vi "EKG Monitor2.vi"() -> ()   [LabVIEW 2010]
uses:
  <instrlib>/niHWS/nihws.llb/niHWS Open File Permissions ID.ctl
  <vilib>/DAQmx/read.llb/DAQmx Read (Analog 1D Wfm NChan NSamp).vi
  <vilib>/DAQmx/create/channels.llb/DAQmx Create Channel (AI-Voltage-Basic).vi
  <vilib>/DAQmx/configure/timing.llb/DAQmx Timing (Sample Clock).vi
  Fear Conditioning/GlobalFear.vi
  <instrlib>/niHWS/nihws.llb/niHWS Write Digital U32.vi
  <instrlib>/niHWS/nihws.llb/niHWS Write Analog DBL.vi
  <instrlib>/niHWS/nihws.llb/niHWS Write Analog WDT.vi
  <vilib>/measure/matone.llb/Extract Single Tone Information N Chan.vi
  <vilib>/daqmx/miscellaneous.llb/DAQmx Fill In Error Info.vi
  Program Files (x86)/National Instruments/LabVIEW 2010/resource/objmgr/daqmx.rc
  <vilib>/measure/NI_MAPro.lvlib
panel:
  out "det Freq":dbl
  out "RAW ECG Signal":waveform(dbl)[](graph)
  in  "# average":dbl=20.0
  out "Shock":bool
  out "Audio":bool
  in  "DPI":dbl=350.0
  out "Cycles \ncompleted":dbl
  in  "stop 2":bool
  in  "Start":bool
  in  "Rate Corrector":bool=TRUE
  out "Skipped":bool
  out "Error Thr":dbl
  out "Threshold":dbl
  in  "HR % Change\nThreshold":dbl(slide)=25.0 scale=0.0..25.0
  out "Detected HR":dynamicdata(graph)
  in  "Mouse Axis":bool
  out "Activity monitor":dynamicdata(graph)
  in  "Activity mouse":refnum<visa-resource-name>
  out "HR":dbl format="%#_4g"
  out "HR":dbl(graph)
  out "Filtered ECG Signal":waveform(dbl)[](graph)
  in  "Recording Path":path
  in  "Record":bool
  in  "stop":bool
  in  "Recording channels":tag
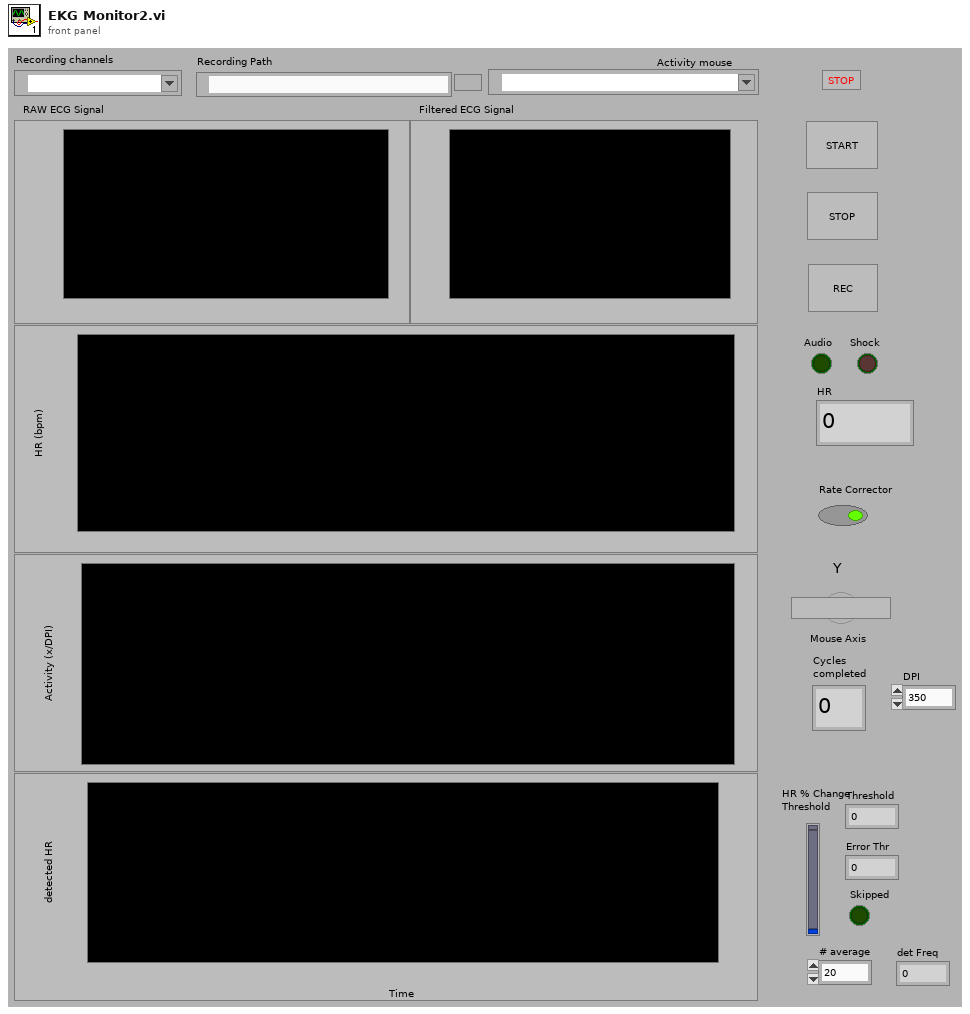
[diagram p1: front panel]
types:
  T1 = typedef "niHWS Open File Permissions ID.ctl" = enum32{"Read Only", "Read/Write Existing", "Read/Write/Create New", "Read/Write/Create New Always"}
  T2 = cluster{"approx freq. (optional)":dbl, "search (+/- % of Fsampl.)":dbl}
  T3 = cluster{"Array":dbl[], "Array 2":dbl[], "Array 3":dbl[], "Array 4":dbl[], "Array 5":dbl[], "Array 6":dbl[], "Array 7":dbl[], "Array 8":dbl[]}
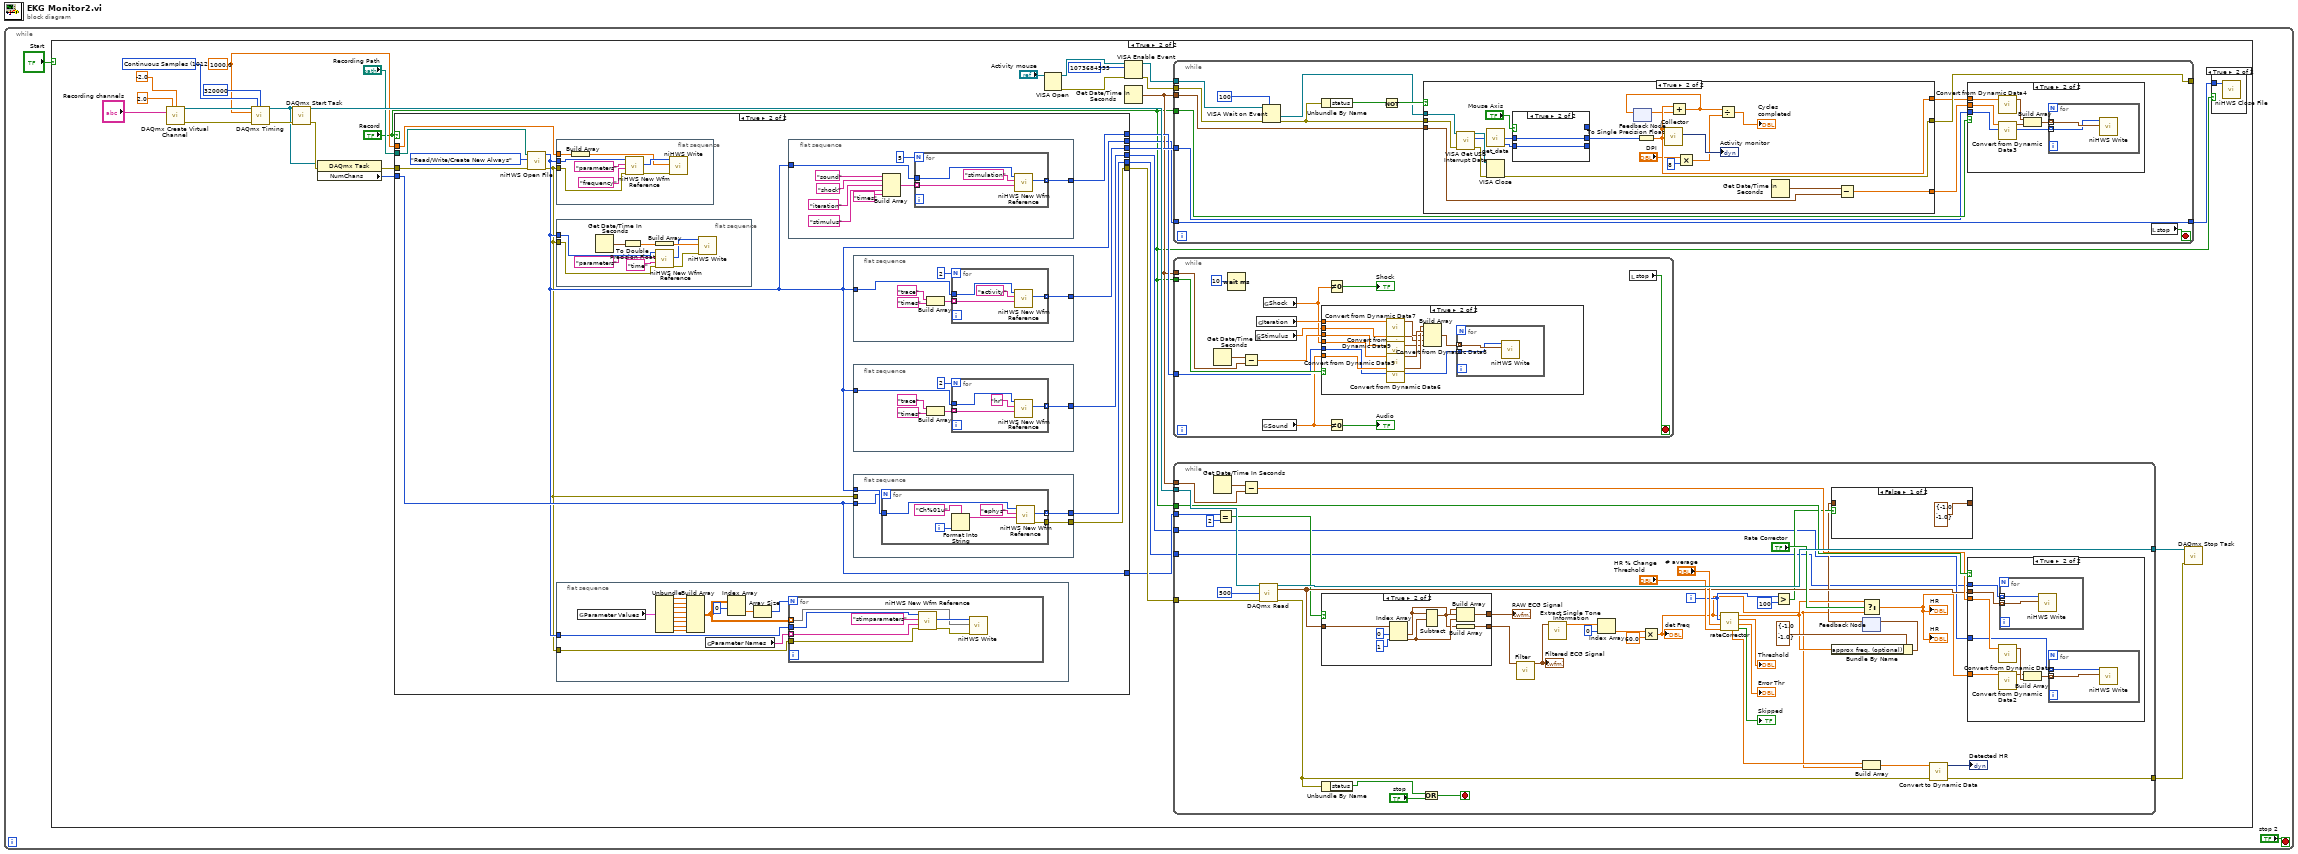
[diagram p0: block diagram]
diagram:
  n1 = while {
    stop <- "stop 2" stop-if-true
    n2 = case shown="True" "Start" {
      frame False {
      }
      frame True {
        w31 = 10123 items=["Finite Samples"=10178, "Continuous Samples"=10123, "Hardware Timed Single Point"=12522] ("sample mode")
        w5 = 1000.0 ("rate")
        n3 = call-poly <vilib>:"DAQmx Create Virtual Channel.vi"("maximum value"=2.0, "minimum value"=-2.0, "physical channels"="Recording channels") -> ("task out"=w32:refnum<k21>, "error out"=w29:errorcluster)  [unwired: 11 in]
        n4 = call-poly <vilib>:"DAQmx Timing.vi"("task/channels in"=w32, "sample mode"=w31, "samples per channel"=320000, "rate"=w5, "error in"=w29) -> ("task out"=w19:refnum<k21>, "error out"=w28:errorcluster)  [unwired: 9 in]
        n5 = call <vilib>:"DAQmx Start Task.vi"("task/channels in"=w19, "error in"=w28) -> ("task out"=w27:refnum<k21>, "error out"=w22:errorcluster)  [unwired: 12 in]
        n6 = property class="DAQmx Task"(reference=w19, error in=w22) -> (error out=w21:errorcluster, "NumChans"=w24:u32)  [unwired: 1 out]
        n7 = case shown="True" "Record" {
          tunnel: w24 -> [w113 w121]
          tunnel: "Recording Path" -> [_ w126]
          tunnel: [w114 w115] -> w20
          tunnel: w21 -> [w114 w124]
          tunnel: [_ w123] -> w12
          tunnel: [_ w122] -> w11
          tunnel: [_ w118] -> w9
          tunnel: [w113 w121] -> w7
          tunnel: [_ w120] -> w6
          tunnel: w5 -> [_ w119]
          tunnel: [_ w116] -> w4
          frame False {
          }
          frame True {
            n8 = call <instrlib>:"niHWS Open File.vi"("error in (no error)"=w124, "permissions (0:read only)"=niHWS_Open_File_Permissions_ID."Read/Write/Create New Always", "file path"=w126) -> ("error out"=w117:errorcluster, "file handle"=w118:u32)  [unwired: 7 in]
            n9 = flat-sequence {
              tunnel: w119 -> [w183]
              tunnel: w117 -> [w182]
              tunnel: w118 -> [w181]
              frame #0 {
                n10 = Build Array(w183) -> (w184:dbl[])
                n11 = call <instrlib>:"niHWS New Wfm Reference.vi"("error in (no error)"=w182, "waveform name (empty)"="frequency" ("group name (empty)"), "group name (empty)"="parameters", "file handle in"=w181) -> ("error out"=w180:errorcluster, "waveform reference"=w187:u32)  [unwired: 5 in, 1 out]
                n12 = call-poly <instrlib>:"niHWS Write.vi"("error in (no error)"=w180, "data"=w184, "waveform reference in"=w187) -> ()  [unwired: 7 in, 2 out]
              }
            }
            n13 = flat-sequence {
              tunnel: w117 -> [w179]
              tunnel: w118 -> [w178]
              frame #0 {
                n14 = Get Date/Time In Seconds() -> (seconds since 1Jan1904=w177:timestamp)
                n15 = To Double Precision Float(number=w177) -> (double precision float=w176:dbl)
                n16 = Build Array(w176) -> (w175:dbl[])
                n17 = call <instrlib>:"niHWS New Wfm Reference.vi"("error in (no error)"=w179, "waveform name (empty)"="time" ("group name (empty)"), "group name (empty)"="parameters", "file handle in"=w178) -> ("error out"=w171:errorcluster, "waveform reference"=w172:u32)  [unwired: 5 in, 1 out]
                n18 = call-poly <instrlib>:"niHWS Write.vi"("error in (no error)"=w171, "data"=w175, "waveform reference in"=w172) -> ()  [unwired: 7 in, 2 out]
              }
            }
            n19 = flat-sequence {
              tunnel: w118 -> [w189]
              tunnel: w117 -> [w188]
              frame #0 {
                n20 = global read "GlobalFear.vi" "Parameter Values"() -> (w190:T3)
                n21 = Unbundle(w190) -> ("Array"=w191:dbl[], "Array 2"=w192:dbl[], "Array 3"=w193:dbl[], "Array 4"=w194:dbl[], "Array 5"=w195:dbl[], "Array 6"=w196:dbl[], "Array 7"=w197:dbl[], "Array 8"=w198:dbl[])
                n22 = Build Array(w191, w192, w193, w194, w195, w196, w197, w198) -> (w202:dbl[][])
                n23 = global read "GlobalFear.vi" "Parameter Names"() -> (w203:string[])
                n24 = Index Array(array=w202, index (row)=0) -> (element=w200:dbl[])  [unwired: 1 in]
                n25 = Array Size(array=w200) -> (size(s)=w199:i32)
                n26 = for {
                  N: w199 -> [_]
                  tunnel: w202 -> [w208] mode=indexing
                  tunnel: w203 -> [w207] mode=indexing
                  tunnel: w189 -> [w206]
                  tunnel: w188 -> [w205]
                  n27 = call <instrlib>:"niHWS New Wfm Reference.vi"("error in (no error)"=w205, "waveform name (empty)"=w207, "group name (empty)"="stimparameters", "file handle in"=w206) -> ("error out"=w204:errorcluster, "waveform reference"=w209:u32)  [unwired: 5 in, 1 out]
                  n28 = call-poly <instrlib>:"niHWS Write.vi"("error in (no error)"=w204, "data"=w208, "waveform reference in"=w209) -> ()  [unwired: 7 in, 2 out]
                }
              }
            }
            n29 = flat-sequence {
              tunnel: [w134] -> w122
              tunnel: w118 -> [w133]
              frame #0 {
                n30 = Build Array("sound" ("format string"), "shock" ("format string"), "iteration" ("format string"), "stimulus" ("format string"), "times") -> (w127:string[])
                n31 = for {
                  N: 5 -> [_]
                  tunnel: [w139] -> w134 mode=indexing
                  tunnel: w133 -> [w137]
                  tunnel: w127 -> [w136] mode=indexing
                  n32 = call <instrlib>:"niHWS New Wfm Reference.vi"("waveform name (empty)"=w136, "group name (empty)"="stimulation", "file handle in"=w137) -> ("waveform reference"=w139:u32)  [unwired: 6 in, 2 out]
                }
              }
            }
            n33 = flat-sequence {
              tunnel: [w155] -> w123
              tunnel: w118 -> [w154]
              frame #0 {
                n34 = Build Array("trace" ("format string"), "times" ("format string")) -> (w150:string[])
                n35 = for {
                  N: 2 -> [_]
                  tunnel: [w159] -> w155 mode=indexing
                  tunnel: w154 -> [w157]
                  tunnel: w150 -> [w156] mode=indexing
                  n36 = call <instrlib>:"niHWS New Wfm Reference.vi"("waveform name (empty)"=w156, "group name (empty)"="activity", "file handle in"=w157) -> ("waveform reference"=w159:u32)  [unwired: 6 in, 2 out]
                }
              }
            }
            n37 = flat-sequence {
              tunnel: [w144] -> w120
              tunnel: w118 -> [w143]
              frame #0 {
                n38 = Build Array("trace" ("format string"), "times" ("format string")) -> (w140:string[])
                n39 = for {
                  N: 2 -> [_]
                  tunnel: [w149] -> w144 mode=indexing
                  tunnel: w143 -> [w147]
                  tunnel: w140 -> [w146] mode=indexing
                  n40 = call <instrlib>:"niHWS New Wfm Reference.vi"("waveform name (empty)"=w146, "group name (empty)"="hr", "file handle in"=w147) -> ("waveform reference"=w149:u32)  [unwired: 6 in, 2 out]
                }
              }
            }
            n41 = flat-sequence {
              tunnel: w121 -> [w162]
              tunnel: w118 -> [w163]
              tunnel: w117 -> [_]
              tunnel: [w161] -> w116
              tunnel: [w160] -> w115
              frame #0 {
                n42 = for {
                  N: w162 -> [_]
                  tunnel: [w165] -> w161 mode=indexing
                  tunnel: [w164] -> w160
                  tunnel: w163 -> [w170]
                  i -> [w168]
                  n43 = Format Into String(format string="Ch%01u", w168) -> (resulting string=w166:string)  [unwired: 2 in, 1 out]
                  n44 = call <instrlib>:"niHWS New Wfm Reference.vi"("waveform name (empty)"=w166, "group name (empty)"="ephys", "file handle in"=w170) -> ("error out"=w164:errorcluster, "waveform reference"=w165:u32)  [unwired: 6 in, 1 out]
                }
              }
            }
          }
        }
        n45 = VISA Open(VISA resource name="Activity mouse") -> (VISA resource name=w18:refnum<visa-resource-name>, error out=w17:errorcluster)  [unwired: 1 in, 3 out]
        n46 = VISA Enable Event(8:w17, 10:u32 1073684535 ("event type"), 11:w18) -> (0:w14:errorcluster, 3:w15:refnum<visa-resource-name>)  [unwired: 1 out]
        n47 = Get Date/Time In Seconds() -> (seconds since 1Jan1904=w10:timestamp)
        n48 = while {
          tunnel: w15 -> [w77]
          tunnel: w14 -> [w76]
          tunnel: w10 -> [w75]
          tunnel: [w69] -> _
          tunnel: "Record" -> [w68]
          tunnel: w12 -> [w65]
          tunnel: w9 -> [w63]
          tunnel: [w63] -> w8
          stop <- w64 stop-if-true
          n49 = VISA Wait on Event(7:u32 100 ("timeout (0)"), 8:w76, 11:w77) -> (0:w70:errorcluster, 1:w71:refnum<visa-resource-name>)  [unwired: 4 out]
          n50 = Unbundle By Name(w70) -> ("status"=w72:bool)
          n51 = Not(x=w72) -> (.not. x?=w73:bool)
          n52 = case shown="True" w73 {
            tunnel: w71 -> [_ w104]
            tunnel: [w86 w103] -> w69
            tunnel: w70 -> [w86 w102]
            tunnel: w75 -> [_ w100]
            tunnel: [_ w93] -> w67
            tunnel: [_ w99] -> w66
            frame False {
            }
            frame True {
              n53 = call <vilib>:"VISA Get USB Interrupt Data.vi"("error in (no error)"=w102, "VISA USB Intr Event"=w104) -> ("error out"=w105:errorcluster, "data buffer"=w101:u8[], "VISA USB Intr Event out"=w106:refnum<visa-resource-name>)  [unwired: 7 out]
              n54 = call "get_data.vi"("data buffer"=w101) -> ("X Value"=w96:i8, "Y Value"=w94:i8)  [unwired: 1 out]
              n55 = VISA Close(VISA resource name=w106, error in (no error)=w105) -> (error out=w103:errorcluster)
              n56 = case shown="True" "Mouse Axis" {
                tunnel: w96 -> [w108 w111]
                tunnel: [w109 w111] -> w95
                tunnel: w94 -> [w109 w110]
                tunnel: [w108 _] -> _
                tunnel: [_ w110] -> _
                frame False {
                }
                frame True {
                }
              }
              n57 = feedback #1() -> (w92:sgl)  [unwired: 1 in]
              n58 = To Single Precision Float(number=w95) -> (single precision float=w93:sgl)
              n59 = call "Collector"("Signals"=w93) -> ("Collected Signals"=→"Activity monitor":dynamicdata)  [unwired: 9 in, 1 out]
              n60 = Add(x=w93, y=w92) -> (x+y=w90:sgl)
              n61 = feedback-in #1(w90) -> ()
              n62 = Multiply(x="DPI", y=8) -> (x*y=w91:dbl)
              n63 = Divide(x=w90, y=w91) -> (x/y=→"Cycles \ncompleted":dbl)
              n64 = Get Date/Time In Seconds() -> (seconds since 1Jan1904=w107:timestamp)
              n65 = Subtract(x=w107, y=w100) -> (x-y=w99:dbl)
            }
          }
          n66 = case shown="True" w68 {
            tunnel: w67 -> [_ w80]
            tunnel: w66 -> [_ w79]
            tunnel: w65 -> [_ w78]
            frame False {
            }
            frame True {
              n67 = call "Convert from Dynamic Data4"("Dynamic Data Type"=w80) -> ("Waveform"=w81:waveform(dbl))  [unwired: 3 in]
              n68 = call "Convert from Dynamic Data3"("Dynamic Data Type"=w79) -> ("Waveform"=w82:waveform(dbl))  [unwired: 3 in]
              n69 = Build Array(w81, w82) -> (w83:waveform(dbl)[])
              n70 = for {
                tunnel: w83 -> [w85] mode=indexing
                tunnel: w78 -> [w84] mode=indexing
                n71 = call-poly <instrlib>:"niHWS Write.vi"("analog waveform"=w85, "waveform reference in"=w84) -> ()  [unwired: 8 in, 2 out]
              }
            }
          }
          n72 = local read "stop"() -> (w64:bool)
        }
        n73 = while {
          tunnel: "Record" -> [w47]
          tunnel: w11 -> [w46]
          tunnel: w10 -> [w44]
          stop <- w48 stop-if-true
          n74 = Get Date/Time In Seconds() -> (seconds since 1Jan1904=w45:timestamp)
          n75 = Wait (ms)(milliseconds to wait=10) -> ()  [unwired: 1 out]
          n76 = Subtract(x=w45, y=w44) -> (x-y=w43:dbl)
          n77 = global read "GlobalFear.vi" "Stimulus"() -> (w36:dbl)
          n78 = global read "GlobalFear.vi" "Iteration"() -> (w42:dbl)
          n79 = global read "GlobalFear.vi" "Sound"() -> (w41:dbl)
          n80 = global read "GlobalFear.vi" "Shock"() -> (w39:dbl)
          n81 = case shown="True" w47 {
            tunnel: w41 -> [_ w57]
            tunnel: w39 -> [_ w56]
            tunnel: w46 -> [_ w55]
            tunnel: w43 -> [_ w53]
            tunnel: w42 -> [_ w52]
            tunnel: w36 -> [_ w49]
            frame False {
            }
            frame True {
              n82 = call "Convert from Dynamic Data7"("Dynamic Data Type"=w52) -> ("Waveform"=w54:waveform(dbl))  [unwired: 3 in]
              n83 = call "Convert from Dynamic Data9"("Dynamic Data Type"=w49) -> ("Waveform"=w50:waveform(dbl))  [unwired: 3 in]
              n84 = call "Convert from Dynamic Data8"("Dynamic Data Type"=w53) -> ("Waveform"=w51:waveform(dbl))  [unwired: 3 in]
              n85 = call "Convert from Dynamic Data5"("Dynamic Data Type"=w56) -> ("Waveform"=w59:waveform(dbl))  [unwired: 3 in]
              n86 = call "Convert from Dynamic Data6"("Dynamic Data Type"=w57) -> ("Waveform"=w58:waveform(dbl))  [unwired: 3 in]
              n87 = Build Array(w58, w59, w54, w50, w51) -> (w60:waveform(dbl)[])
              n88 = for {
                tunnel: w60 -> [w62] mode=indexing
                tunnel: w55 -> [w61] mode=indexing
                n89 = call-poly <instrlib>:"niHWS Write.vi"("analog waveform"=w62, "waveform reference in"=w61) -> ()  [unwired: 8 in, 2 out]
              }
            }
          }
          n90 = Not Equal To 0?(x=w39) -> (x != 0?=→"Shock":bool)
          n91 = Not Equal To 0?(x=w41) -> (x != 0?=→"Audio":bool)
          n92 = local read "stop"() -> (w48:bool)
        }
        n93 = while {
          tunnel: w27 -> [w253]
          tunnel: w20 -> [w252]
          tunnel: [w251] -> w26
          tunnel: [w249] -> w25
          tunnel: "Record" -> [w245]
          tunnel: w10 -> [w239]
          tunnel: w7 -> [w218]
          tunnel: w6 -> [w212]
          tunnel: w4 -> [w211]
          i -> [w216]
          stop <- w246 stop-if-true
          n94 = Get Date/Time In Seconds() -> (seconds since 1Jan1904=w240:timestamp)
          n95 = Equal?(x=w218, y=2) -> (x = y?=w219:bool)
          n96 = Subtract(x=w240, y=w239) -> (x-y=w238:dbl)
          n97 = call-poly <vilib>:"DAQmx Read.vi"("task/channels in"=w253, "number of samples per channel"=500, "error in"=w252) -> ("task out"=w251:refnum<k21>, "data"=w231:waveform(dbl)[], "error out"=w249:errorcluster)  [unwired: 10 in]
          n98 = case shown="True" w219 {
            tunnel: w231 -> [w256 w262]
            tunnel: [w256 w261] -> w230
            tunnel: [w256 w260] -> w221
            frame False {
            }
            frame True {
              n99 = Index Array(array=w262, index #1=0 ("index"), index #2=1 ("index")) -> (element #1=w258:waveform(dbl), element #2=w259:waveform(dbl))
              n100 = Subtract(1:w259, 2:w258) -> (0:w257:waveform(dbl))  [unwired: 1 in, 1 out]
              n101 = Build Array(w257, w258, w259) -> (w260:waveform(dbl)[])
              n102 = Build Array(w257) -> (w261:waveform(dbl)[])
            }
          }
          "RAW ECG Signal" <- w221
          n103 = Unbundle By Name(w249) -> ("status"=w248:bool)
          n104 = Or(x=w248, y="stop") -> (x .or. y?=w246:bool)
          n105 = call "Filter"("input signals"=w230) -> ("filtered data"=w241:waveform(dbl)[])  [unwired: 17 in, 1 out]
          "Filtered ECG Signal" <- w241
          n106 = call-poly <vilib>:"Extract Single Tone Information.vi"("time signals in"=w241) -> ("detected frequencies"=w244:dbl[])  [unwired: 5 in, 5 out]
          n107 = Index Array(array=w244, index=0) -> (element=w224:dbl)
          n108 = Multiply(x=w224, y=60.0) -> (x*y=w213:dbl)
          "det Freq" <- w213
          n109 = call "rateCorrector.vi"("threshold"="HR % Change\nThreshold", "intergration"="# average", "count"=w216, "HR"=w213) -> ("skipped"=→"Skipped":bool, "error count"=→"Error Thr":dbl, "actual threshold"=→"Threshold":dbl, "HR"=w222:dbl, "Raw corr"=w226:dbl)  [unwired: 3 in]
          n110 = Greater?(x=w216, y=100 ("index")) -> (0:w215:bool)
          n111 = Bundle By Name(cluster=T2 {"approx freq. (optional)"=-1.0, "search (+/- % of Fsampl.)"=-1.0} ("advanced search"), "approx freq. (optional)"=w222) -> (w223:T2)
          n112 = Select(t=w222, s="Rate Corrector", f=w213) -> (s? t:f=w229:dbl)
          "HR" <- w229
          "HR" <- w229
          n113 = feedback-in #2(w223) -> ()
          n114 = feedback #2() -> (w214:T2)  [unwired: 1 in]
          n115 = case shown="False" w215 {
            tunnel: [T2 {"approx freq. (optional)"=-1.0, "search (+/- % of Fsampl.)"=-1.0} ("advanced search") w255] -> _
            tunnel: w214 -> [_ w255]
            frame False {
            }
            frame True {
            }
          }
          n116 = Build Array(w226, w213) -> (w228:dbl[])
          n117 = call "Convert to Dynamic Data"("Array"=w228) -> ("Dynamic Data Type"=→"Detected HR":dynamicdata)  [unwired: 3 in]
          n118 = case shown="True" w245 {
            tunnel: w231 -> [_ w272]
            tunnel: w238 -> [_ w268]
            tunnel: w229 -> [_ w267]
            tunnel: w212 -> [_ w266]
            tunnel: w211 -> [_ w265]
            frame False {
            }
            frame True {
              n119 = call "Convert from Dynamic Data"("Dynamic Data Type"=w268) -> ("Waveform"=w271:waveform(dbl))  [unwired: 3 in]
              n120 = call "Convert from Dynamic Data2"("Dynamic Data Type"=w267) -> ("Waveform"=w270:waveform(dbl))  [unwired: 3 in]
              n121 = for {
                tunnel: w272 -> [w276] mode=indexing
                tunnel: w265 -> [w275] mode=indexing
                n122 = call-poly <instrlib>:"niHWS Write.vi"("analog waveform"=w276, "waveform reference in"=w275) -> ()  [unwired: 8 in, 2 out]
              }
              n123 = Build Array(w270, w271) -> (w269:waveform(dbl)[])
              n124 = for {
                tunnel: w269 -> [w274] mode=indexing
                tunnel: w266 -> [w273] mode=indexing
                n125 = call-poly <instrlib>:"niHWS Write.vi"("analog waveform"=w274, "waveform reference in"=w273) -> ()  [unwired: 8 in, 2 out]
              }
            }
          }
        }
        n126 = call <vilib>:"DAQmx Stop Task.vi"("task/channels in"=w26, "error in"=w25) -> ()  [unwired: 12 in, 2 out]
        n127 = case shown="True" "Record" {
          tunnel: w8 -> [_ w112]
          frame False {
          }
          frame True {
            n128 = call <instrlib>:"niHWS Close File.vi"("file handle"=w112) -> ()  [unwired: 10 in, 1 out]
          }
        }
      }
    }
  }
